vi "main.vi"() -> ()   [LabVIEW 2021]
uses:
  <vilib>/Analysis/baseanly.llb/Mean (DBL).vi
  <vilib>/Utility/file.llb/Read Delimited Spreadsheet (DBL).vi
  <vilib>/Analysis/NI_AALBase.lvlib
panel:
  out "sum":dbl
  out "mean":dbl format="%0.5f"
  out "Histogram Graph":T1(graph)
  out "size(s) 2":i32
  out "Array":dbl[](array[numeric])
  out "flancos negativos":i32[](array[numeric])
  out "flancos positivos":i32[](array[numeric])
  out "size(s)":i32
  in  "Control de umbral":dbl
  out "Curva de potencia":cluster{"all rows":dbl[], "all rows":dbl[]}[](graph)
  in  "error in":errorcluster
  in  "file (use dialog)":path
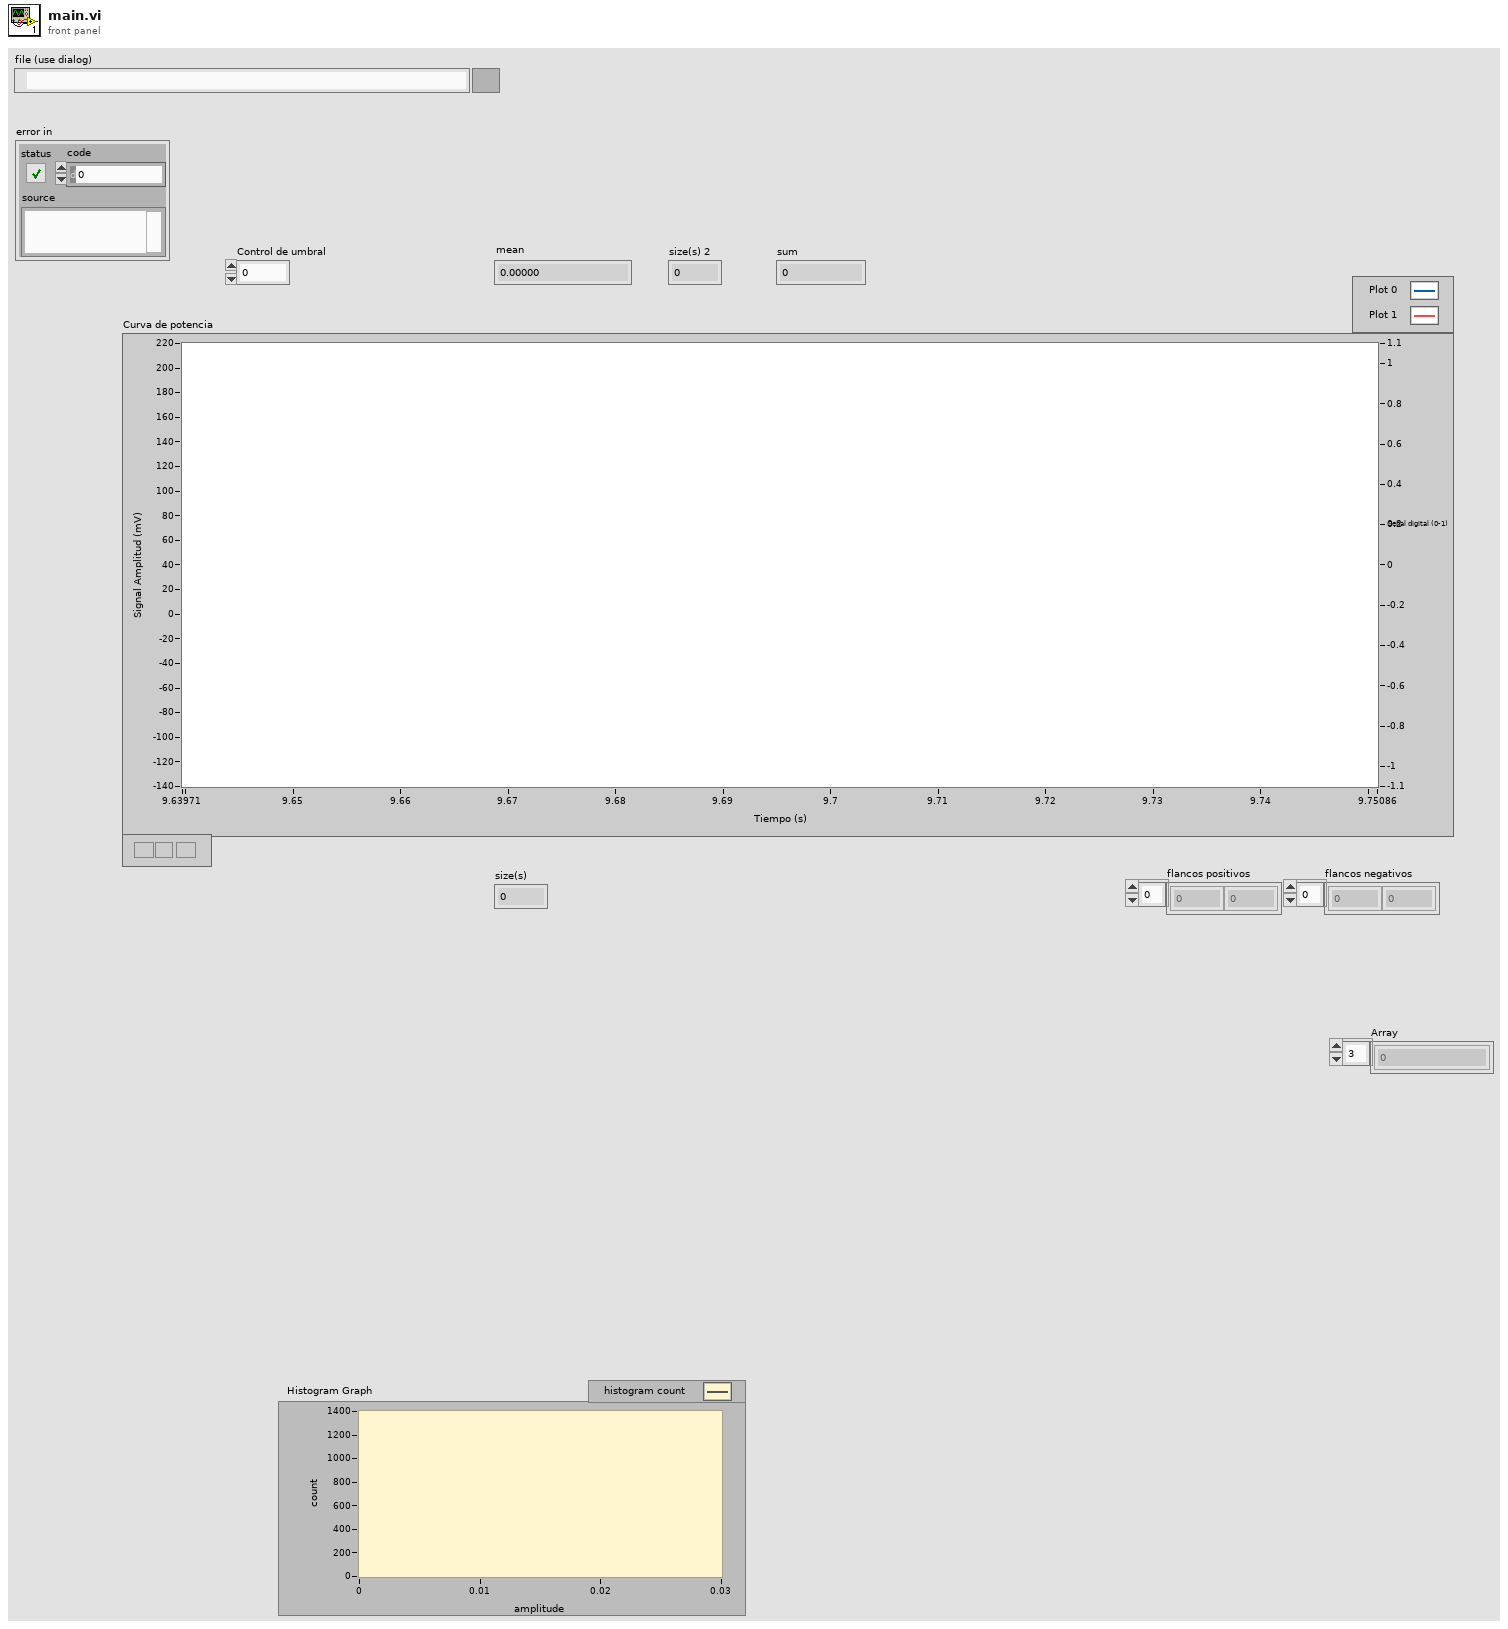
[diagram p1: front panel]
types:
  T1 = cluster{"X Values":dbl[], "Histogram: h(x)":i32[]}
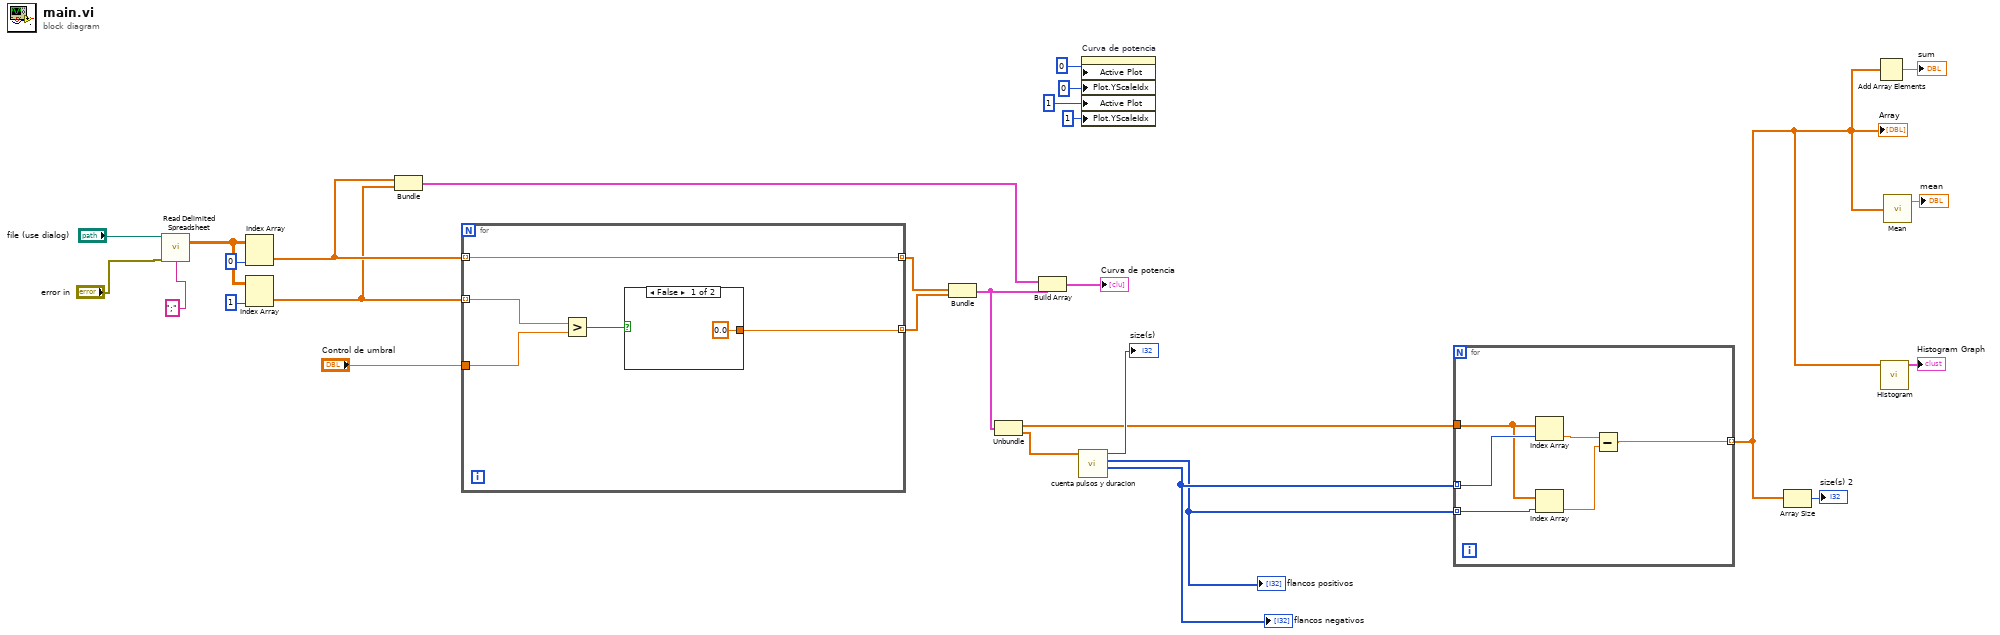
[diagram p0: block diagram]
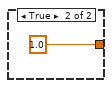
[diagram p2: hidden frame]
diagram:
  n1 = call-poly <vilib>:"Read Delimited Spreadsheet.vi"("file path (dialog if empty)"="file (use dialog)", "error in (no error)"="error in", "delimiter (\\t)"=";" ("delimiter (\\t)")) -> ("all rows"=w25:dbl[][])  [unwired: 7 in, 5 out]
  n2 = Index Array(array=w25, index (col)=0 ("disabled index (col)")) -> (element=w22:dbl[])  [unwired: 1 in]
  n3 = Index Array(array=w25, index (col)=1 ("disabled index (col)")) -> (element=w21:dbl[])  [unwired: 1 in]
  n4 = Bundle("all rows"=w22, "all rows"=w21) -> (w17:cluster{"all rows":dbl[], "all rows":dbl[]})  [unwired: 1 in]
  n5 = for {
    tunnel: w22 -> [w33] mode=indexing
    tunnel: w21 -> [w32] mode=indexing
    tunnel: [w33] -> w19 mode=indexing
    tunnel: "Control de umbral" -> [w31]
    tunnel: [w29] -> w18 mode=indexing
    n6 = Greater?(x=w32, y=w31) -> (0:w30:bool)
    n7 = case shown="False" w30 {
      tunnel: [0.0 ("Numeric") 1.0 ("Numeric")] -> w29
      frame False {
      }
      frame True {
      }
    }
  }
  n8 = Bundle(w19, w18) -> (w11:cluster{dbl[], dbl[]})  [unwired: 1 in]
  n9 = Unbundle(w11) -> (w8:dbl[], w10:dbl[])
  n10 = Build Array(w17, w11) -> (→"Curva de potencia":cluster{"all rows":dbl[], "all rows":dbl[]}[])
  n11 = call "cuenta pulsos y duracion.vi"("Array 2"=w10) -> ("flancos negativos"=w7:i32[], "flancos positivos"=w6:i32[], "size(s)"=→"size(s)":i32)  [unwired: 8 in]
  "flancos positivos" <- w6
  "flancos negativos" <- w7
  n12 = property on="Curva de potencia" class="XYGraph (strict)"("Active Plot"=u32 0, "Plot.YScaleIdx"=u32 0 ("Active Plot"), "Active Plot"=u32 1, "Plot.YScaleIdx"=u32 1 ("Plot.Y Scale Index")) -> ()  [unwired: 2 in, 2 out]
  n13 = for {
    tunnel: w8 -> [w39]
    tunnel: w7 -> [w41] mode=indexing
    tunnel: w6 -> [w38] mode=indexing
    tunnel: [w36] -> w2 mode=indexing
    n14 = Index Array(array=w39, index=w41) -> (element=w40:dbl)
    n15 = Index Array(array=w39, index=w38) -> (element=w37:dbl)
    n16 = Subtract(x=w40, y=w37) -> (x-y=w36:dbl)
  }
  "Array" <- w2
  n17 = Array Size(array=w2) -> (size(s)=→"size(s) 2":i32)
  n18 = Add Array Elements(numeric array=w2) -> (sum=→"sum":dbl)
  n19 = call <vilib>:"Histogram.vi"("X"=w2) -> ("Histogram Graph"=→"Histogram Graph":T1)  [unwired: 7 in, 3 out]
  n20 = call-poly <vilib>:"Mean.vi"("X"=w2) -> ("mean"=→"mean":dbl)  [unwired: 1 out]
